vi "Decode Charging State.vi"(11 "Numeric":u8) -> (3 "Charging State":T1(ring))   [LabVIEW 2015]
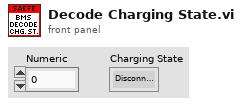
[diagram p1: front panel]
types:
  T1 = enum16{"Disconnected", "Pre-charging", "Main Charging", "Balancing", "Charging Finished OK", "Charging Error"}
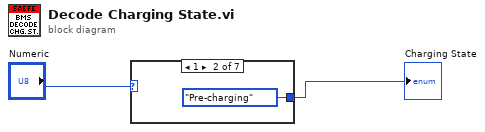
[diagram p0: block diagram]
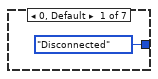
[diagram p2: hidden frame]
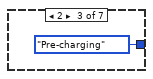
[diagram p3: hidden frame]
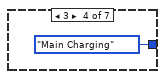
[diagram p4: hidden frame]
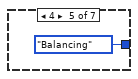
[diagram p5: hidden frame]
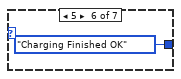
[diagram p6: hidden frame]
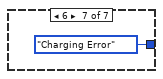
[diagram p7: hidden frame]
diagram:
  n1 = case shown="1" "Numeric" {
    tunnel: [T1."Disconnected" ("Charging State") T1."Pre-charging" ("Charging State") T1."Pre-charging" ("Charging State") T1."Main Charging" ("Charging State") T1."Balancing" ("Charging State") T1."Charging Finished OK" ("Charging State") T1."Charging Error" ("Charging State")] -> w2
    frame 0, Default {
    }
    frame 1 {
    }
    frame 2 {
    }
    frame 3 {
    }
    frame 4 {
    }
    frame 5 {
    }
    frame 6 {
    }
  }
  "Charging State" <- w2
